vi "trace_property_ui_sub.vi"(5 "trace idx global":u32, 7 "properties ui":string[](array[string]), 11 "error in (no error)":errorcluster) -> (8 "properties":T1(array[cluster]), 10 "property":cluster{"property":string, "property value":u32}, 15 "error out":errorcluster)   [LabVIEW 2010, in "OSA.lvclass"]
uses:
  OSA.lvclass
  FTSLib.dll
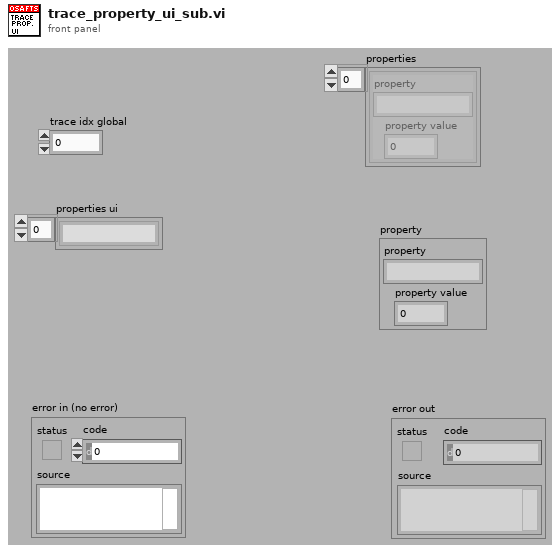
[diagram p1: front panel]
types:
  T1 = cluster{"property":string, "property value":u32}[]
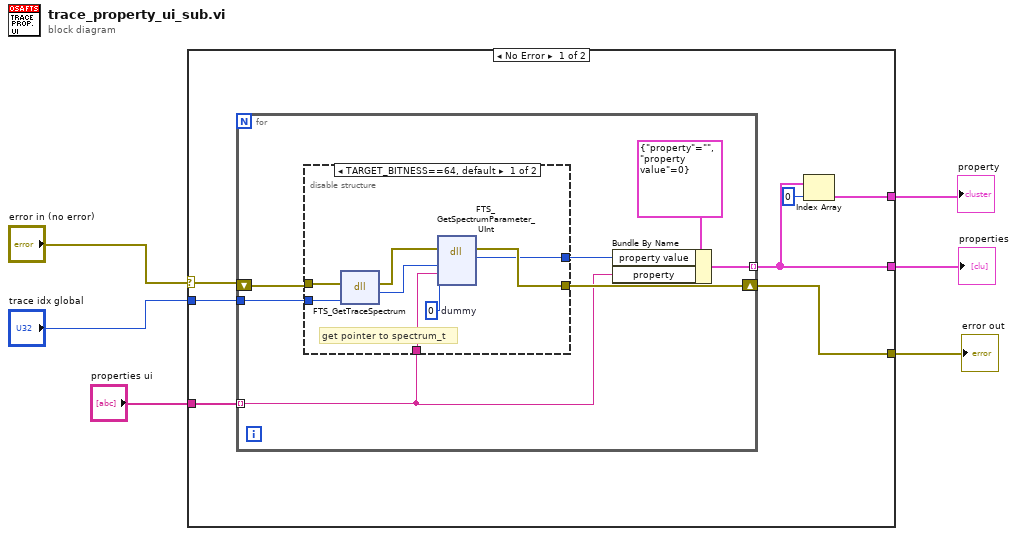
[diagram p0: block diagram]
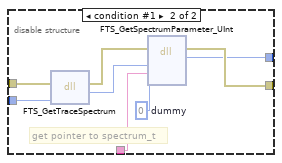
[diagram p2: hidden frame]
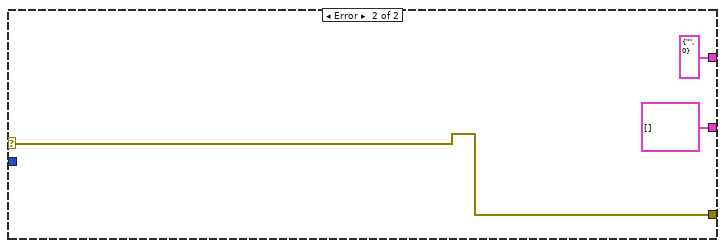
[diagram p3: hidden frame]
diagram:
  n1 = case shown="No Error" "error in (no error)" {
    selector: "error in (no error)" -> [w7 w37]
    tunnel: "properties ui" -> [w13 _]
    tunnel: "trace idx global" -> [w12 _]
    tunnel: [w11 T1 []] -> w4
    tunnel: [w9 cluster{"property":string, "property value":u32} {"property"="", "property value"=0}] -> w1
    tunnel: [w8 w37] -> w3
    frame No Error {
      n2 = for {
        shift-right: [w20] -> w8
        shift-left: w7 -> [w19]
        tunnel: w12 -> [w18]
        tunnel: w13 -> [w15] mode=indexing
        tunnel: [w16] -> w11 mode=indexing
        n3 = disable-structure shown="TARGET_BITNESS==64, default" {
          disable-tunnel: w18 -> [w28 w32]
          disable-tunnel: w15 -> [w27 w31]
          disable-tunnel: w19 -> [w24 w33]
          disable-tunnel: [w23 w30] -> w20
          disable-tunnel: [w21 w29] -> w14
          frame condition #0 (active) {
            w22 = u32 0  # dummy
            # "get pointer to spectrum_t"
            n4 = dll-call lib="FTSLib.dll" fn="FTS_GetTraceSpectrum"(error in=w24, "traceIdx"=w28) -> (error out=w25:errorcluster, "spectrum_t_pointer"=w26:u64)  [unwired: 3 in, 1 out]
            n5 = dll-call lib="FTSLib.dll" fn="FTS_GetSpectrumParameter_UInt"(error in=w25, "spectrum_t_pointer"=w26, "parameter_name"=w27, "array_index"=w22) -> (error out=w23:errorcluster, "parameter"=w21:u32)  [unwired: 5 in, 1 out]
          }
          frame condition #1 {
            w34 = u32 0  # dummy
            # "get pointer to spectrum_t"
            n6 = dll-call lib="FTSLib.dll" fn="FTS_GetTraceSpectrum"(error in=w33, "traceIdx"=w32) -> (error out=w35:errorcluster, "spectrum_t_pointer"=w36:u32)  [unwired: 3 in, 1 out]
            n7 = dll-call lib="FTSLib.dll" fn="FTS_GetSpectrumParameter_UInt"(error in=w35, "spectrum_t_pointer"=w36, "parameter_name"=w31, "array_index"=w34) -> (error out=w30:errorcluster, "parameter"=w29:u32)  [unwired: 5 in, 1 out]
          }
        }
        n8 = Bundle By Name(cluster=cluster{"property":string, "property value":u32} {"property"="", "property value"=0}, "property value"=w14, "property"=w15) -> (w16:cluster{"property":string, "property value":u32})
      }
      n9 = Index Array(array=w11, index=0) -> (element=w9:cluster{"property":string, "property value":u32})
    }
    frame Error {
    }
  }
  "properties" <- w4
  "property" <- w1
  "error out" <- w3
